vi "写入-PC总客户端集.vi"(8 "error in (no error)":errorcluster caption="错误输入（无错误）", 10 "PC总客户端集":refnum<class "PC总客户端.lvclass">[](array[class]), 11 "客户单位输入":refnum<class "客户单位.lvclass">) -> (0 "error out":errorcluster caption="错误输出", 3 "客户单位输出":refnum<class "客户单位.lvclass">)   [LabVIEW 2013, in "客户单位.lvclass"]
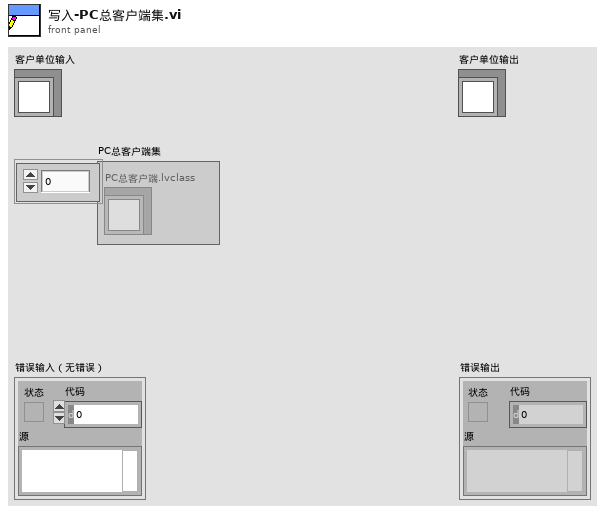
[diagram p1: front panel]
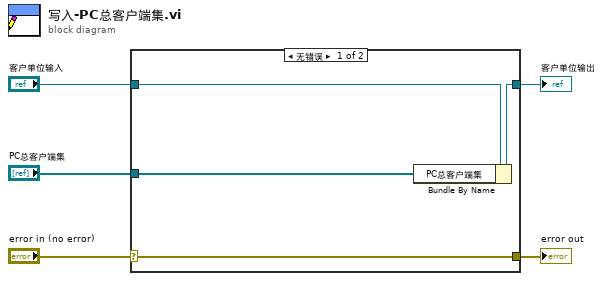
[diagram p0: block diagram]
diagram:
  n1 = case shown="无错误" "error in (no error)" {
    selector: "error in (no error)" -> [w9 w10]
    tunnel: [w9 w10] -> w4
    tunnel: [w7 w11] -> w2
    tunnel: "客户单位输入" -> [w8 w11]
    tunnel: "PC总客户端集" -> [w6 _]
    frame No Error {
      n2 = Bundle By Name(cluster=w8, "PC总客户端集"=w6) -> (w7:refnum<class "客户单位.lvclass">)
    }
    frame Error {
    }
  }
  "error out" <- w4
  "客户单位输出" <- w2
